vi "InsertEventCodes.vi"(0 "reference in":refnum<class "Logger.lvclass">, 11 "error in (no error)":errorcluster) -> (4 "reference out":refnum<class "Logger.lvclass">, 14 "dt (ms)":u32, 15 "error out":errorcluster)   [LabVIEW 2019, in "Logger.lvclass"]
uses:
  Logger.lvclass
  EventCode.ctl
  Logger.lvclass/Logger.ctl
  392f7031-4897-4389-b682-77fa04bcb28f.vi
  9e415a43-db33-4f06-8781-9fdd0a489df8.vi
  DatabaseInterface_class/DatabaseInterface.lvclass
panel:
  in  "EventCode":T1=enum."DI_RAW_HI"
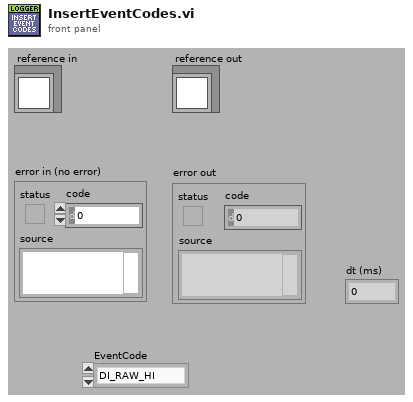
[diagram p1: front panel]
types:
  T1 = typedef "Logger.lvclass/EventCode.ctl" = enum16{"DI_EU_LO", "DI_EU_HI", "DIO_LO", "DIO_HI", "DI_RAW_LO", "DI_RAW_HI", "DO_LO", "DO_HI", "DA_OK", "DA_ALARM", "AA_HI", "AA_HIHI", "AA_LO", "AA_LOLO", "AA_OK", "CMD", "OUT_OF_RANGE_OK", "OUT_OF_RANGE_LO", "OUT_OF_RANGE_HI", "CONFIG", "DI_LO", "DI_HI"}
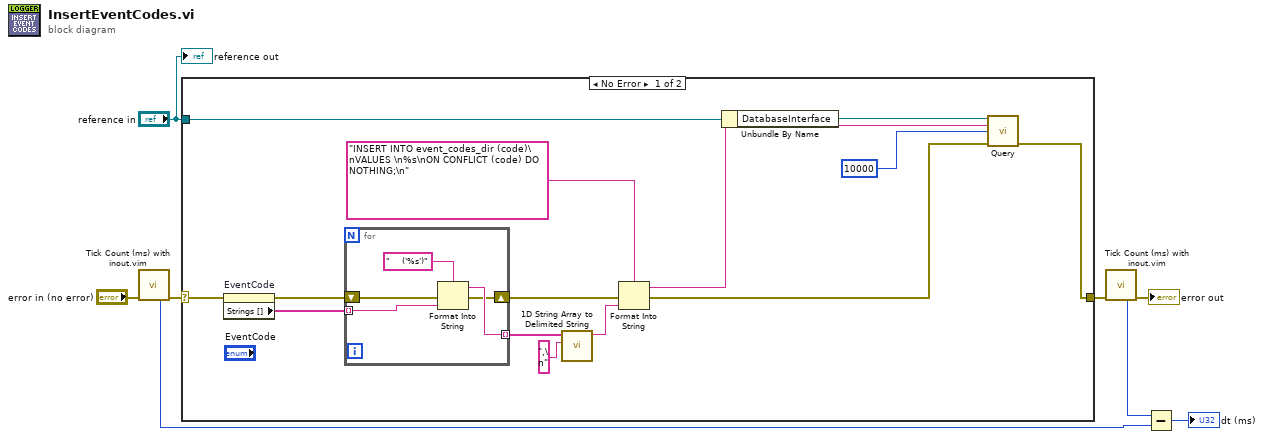
[diagram p0: block diagram]
diagram:
  n1 = call "Tick Count (ms) with inout.vim"("in"="error in (no error)") -> ("millisecond timer value dub"=w3:u32, "out"=w2:errorcluster)  [unwired: 12 in, 1 out]
  n2 = case shown="No Error" w2 {
    selector: w2 -> [w11 w28]
    tunnel: [w10 w28] -> w7
    tunnel: "reference in" -> [w9 _]
    frame No Error {
      n3 = property on="EventCode" class="Enum (strict)"(error in=w11) -> (error out=w13:errorcluster, "Strings []"=w12:string[])  [unwired: 1 in, 1 out]
      n4 = for {
        tunnel: w12 -> [w27] mode=indexing
        tunnel: [w25] -> w22 mode=indexing
        shift-right: [w24] -> w20
        shift-left: w13 -> [w23]
        n5 = Format Into String(format string="    ('%s')", error in=w23, w27) -> (resulting string=w25:string, error out=w24:errorcluster)  [unwired: 1 in]
      }
      n6 = call <vilib>:"1D String Array to Delimited String.vi"("delimiter"=",\n", "string array"=w22) -> ("delimited string"=w17:string)  [unwired: 9 in]
      n7 = Format Into String(format string="INSERT INTO event_codes_dir (code)\nVALUES \n%s\nON CONFLICT (code) DO NOTHING;\n", error in=w20, w17) -> (resulting string=w16:string, error out=w19:errorcluster)  [unwired: 1 in]
      n8 = Unbundle By Name(w9) -> ("DatabaseInterface"=w15:refnum<class "DatabaseInterface.lvclass">)
      n9 = call-dynamic "Query.vi"("reference in"=w15, "Query"=w16, "Timeout"=10000, "error in (no error)"=w19) -> ("error out"=w10:errorcluster)  [unwired: 9 in, 2 out]
    }
    frame Error {
    }
  }
  n10 = call "Tick Count (ms) with inout.vim"("in"=w7) -> ("millisecond timer value dub"=w5:u32, "out"=→"error out":errorcluster)  [unwired: 12 in, 1 out]
  n11 = Subtract(x=w5, y=w3) -> (x-y=→"dt (ms)":u32)
  "reference out" <- "reference in"
